vi "17.2 Particle Classification-Grayscale.vi"() -> ()   [LabVIEW 2016]
doc: "This example shows how to use the classification VIs in NI Vision.\n\nClassification quickly identifies and classifies unknown objects in inspection images. First, use the Classification Training Interface to teach your application the types, or classes, of objects you want to classify. The Classification Training Interface creates a classifier file, which you then use to classify unknown objects into one of the classes you trained."
uses:
  <vilib>/vision/NI_Vision_Development_Module.lvlib
panel:
  out "Scores":T1(array[cluster])
  out "Image":T2(plugin-control)
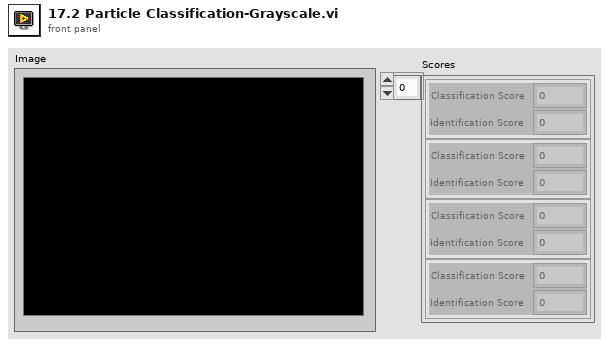
[diagram p1: front panel]
types:
  T1 = cluster{"Classification Score":sgl, "Identification Score":sgl}[]
  T2 = typedef "IMAQ Image.ctl" = refnum<image>
  T3 = typedef "IMAQ Classifier Session.ctl" = refnum<k1>
  T4 = typedef "ROI Descriptor" = cluster{"Global Rectangle":i32[], "Contours":cluster{"ID":enum32{"External", "Internal"}, "Type":u32, "Coordinates":i32[]}[]}
  T5 = cluster{"Classification Score":sgl, "Identification Score":sgl}
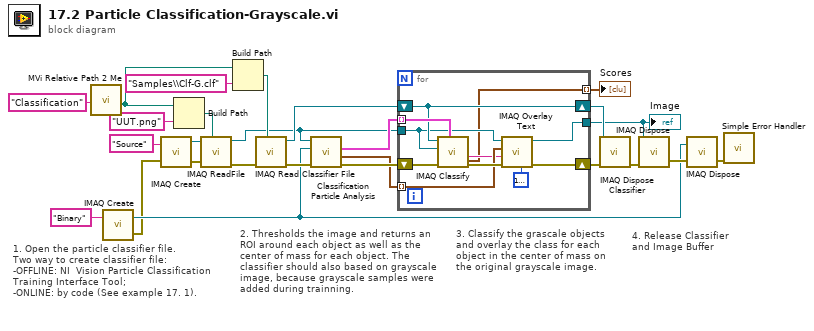
[diagram p0: block diagram]
diagram:
  # "4. Release Classifier and Image Buffer"
  # "1. Open the particle classifier file. \nTwo way to create classifier file:\n-OFFLINE: NI  Vision Particle Classification Training Interface Tool;\n-ONLINE: by code (See example 17. 1)."
  # "3. Classify the grascale objects and overlay the class for each object in the center of mass on the original grayscale image."
  # "2. Thresholds the image and returns an ROI around each object as well as the center of mass for each object. The classifier should also based on grayscale image, because grayscale samples were added during trainning."
  n1 = call "MVi Relative Path 2 Me.vi"("Relative Path"="Classification" ("name or relative path")) -> ("Appended Dir"=w4:path)  [unwired: 5 in, 1 out]
  n2 = call "IMAQ Create"("Image Name"="Binary") -> ("Src"=w11:T2, "error out"=w10:errorcluster)  [unwired: 3 in, 1 out]
  n3 = call "IMAQ Create"("Image Name"="Source", "error in (no error)"=w10) -> ("Src"=w19:T2, "error out"=w18:errorcluster)  [unwired: 2 in, 1 out]
  n4 = Build Path(base path=w4, name or relative path="UUT.png") -> (appended path=w6:path)
  n5 = call "IMAQ ReadFile"("File Path"=w6, "error in (no error)"=w18, "Image"=w19) -> ("error out"=w20:errorcluster, "Image Out"=w3:T2)  [unwired: 4 in, 3 out]
  n6 = Build Path(base path=w4, name or relative path="Samples\\Clf-G.clf") -> (appended path=w21:path)
  n7 = call "IMAQ Read Classifier File"("File Path"=w21, "error in (no error)"=w20) -> ("error out"=w16:errorcluster, "Classifier Session"=w8:T3)  [unwired: 2 in, 6 out]
  n8 = call "Classification Particle Analysis.vi"("error in (no error)"=w16, "Image Dest"=w11, "Image Source"=w3) -> ("error out"=w26:errorcluster, "Center of Masses"=w25:cluster{"X":dbl, "Y":dbl}[], "ROIs"=w24:T4[])  [unwired: 5 in, 1 out]
  n9 = for {
    tunnel: w24 -> [w36] mode=indexing
    tunnel: w25 -> [w33] mode=indexing
    shift-right: [w35] -> w15
    shift-left: w8 -> [w35]
    shift-right: [w32] -> w14
    shift-left: w26 -> [w37]
    tunnel: w3 -> [w28]
    tunnel: [w30] -> w2
    tunnel: [w27] -> w1 mode=indexing
    n10 = call "IMAQ Classify"("ROI Descriptor"=w36, "error in (no error)"=w37, "Image"=w28, "Classifier Session"=w35) -> ("error out"=w34:errorcluster, "Class"=w29:string, "Scores"=w27:T5)  [unwired: 5 out]
    n11 = call "IMAQ Overlay Text"("BG Color (Transparent)"=u32 16777226, "error in (no error)"=w34, "String"=w29, "Origin"=w33, "Image"=w28) -> ("error out"=w32:errorcluster, "Image Out"=w30:T2)  [unwired: 5 in]
  }
  "Image" <- w2
  "Scores" <- w1
  n12 = call "IMAQ Dispose Classifier"("error in (no error)"=w14, "Classifier Session"=w15) -> ("error out"=w13:errorcluster)  [unwired: 9 out]
  n13 = call "IMAQ Dispose"("Image"=w2, "error in (no error)"=w13) -> ("error out"=w12:errorcluster)  [unwired: 1 in, 3 out]
  n14 = call "IMAQ Dispose"("Image"=w11, "error in (no error)"=w12) -> ("error out"=w9:errorcluster)  [unwired: 1 in, 3 out]
  n15 = call <vilib>:"Simple Error Handler.vi"("error in (no error)"=w9) -> ()  [unwired: 4 in, 5 out]
